vi "HOST_laser.vi"() -> ()   [LabVIEW 2018]
uses:
  <vilib>/rvi/interface/nirviOpenFPGA/nirviOpenFPGA.xnode
  <vilib>/rvi/interface/nirviMethod/nirviMethod.xnode
  <vilib>/FPGAPlugInAG/Dynamic/niLvFpga_Reset_Dynamic.vi
  <vilib>/FPGAPlugInAG/Dynamic/niLvFpga_Run_Dynamic.vi
  <vilib>/rvi/interface/nirviReadWriteControl/nirviReadWriteControl.xnode
  <vilib>/rvi/interface/nirviCloseFPGA/nirviCloseFPGA.xnode
  NiFpgaLv.dll
  <vilib>/Utility/error.llb/Error Cluster From Error Code.vi
  <vilib>/rvi/interface/Simulation/niFpgaSimulationCallBeginRW.vi
  <vilib>/rvi/errors/niLvFpgaAdjustHostInterfaceError.vi
  <vilib>/FPGAPlugInAG/Dynamic/niLvFpga_Close_Dynamic.vi
  FPGA Bitfiles/iCLNGNQI_FPGATarget_Target_OrC3no1FGAk.lvbitx
  <vilib>/FPGAPlugInAG/PXI-7841R/niLvFpga_Open_PXI-7841R.vi
  <vilib>/rvi/interface/common/dynamic/niFpgaDynamicAddResources.vi
  <vilib>/userdefined/High Color/nirio_resource_hc.ctl
panel:
  in  "Прошивка":bool
  in  "СТОП":bool
  out "Сбои":i32
  in  "resource name":T1="PXI1Slot6"
  in  "Сверочный массив":bool[][](array[boolean])=[[FALSE, FALSE, FALSE, FALSE, FALSE, TRUE, FALSE, TRUE], [FALSE, FALSE, FALSE, FALSE, FALSE, TRUE, FALSE, TRUE], [FALSE, FALSE, FALSE, FALSE, FALSE, FALSE, TRUE, TRUE], [FALSE, FALSE, FALSE, FALSE, FALSE, FALSE, TRUE, TRUE], [FALSE, FALSE, FALSE, FALSE, FALSE, FALSE, TRUE, TRUE], [FALSE, FALSE, FALSE, FALSE, FALSE, FALSE, TRUE, TRUE], [FALSE, FALSE, FALSE, FALSE, FALSE, TRUE, FALSE, TRUE], [TRUE, FALSE, FALSE, FALSE, FALSE, FALSE, FALSE, TRUE], [FALSE, TRUE, TRUE, FALSE, TRUE, FALSE, FALSE, TRUE]]
  in  "На чтение":bool[][](array[boolean])=[[FALSE, FALSE, FALSE, FALSE, FALSE, FALSE, FALSE, FALSE, FALSE, FALSE, FALSE, FALSE, FALSE, FALSE, FALSE, FALSE, FALSE, TRUE, FALSE, TRUE, FALSE, FALSE, FALSE, TRUE], [FALSE, FALSE, FALSE, FALSE, FALSE, FALSE, FALSE, FALSE, TRUE, FALSE, FALSE, FALSE, FALSE, FALSE, FALSE, FALSE, FALSE, TRUE, FALSE, TRUE, FALSE, FALSE, FALSE, TRUE], [FALSE, FALSE, FALSE, FALSE, FALSE, FALSE, FALSE, FALSE, FALSE, TRUE, FALSE, FALSE, FALSE, FALSE, FALSE, FALSE, FALSE, TRUE, FALSE, TRUE, FALSE, FALSE, FALSE, TRUE], [FALSE, FALSE, FALSE, FALSE, FALSE, FALSE, FALSE, FALSE, TRUE, TRUE, FALSE, FALSE, FALSE, FALSE, FALSE, FALSE, FALSE, TRUE, FALSE, TRUE, FALSE, FALSE, FALSE, TRUE], [FALSE, FALSE, FALSE, FALSE, FALSE, FALSE, FALSE, FALSE, FALSE, FALSE, TRUE, FALSE, FALSE, FALSE, FALSE, FALSE, FALSE, TRUE, FALSE, TRUE, FALSE, FALSE, FALSE, TRUE], [FALSE, FALSE, FALSE, FALSE, FALSE, FALSE, FALSE, FALSE, TRUE, FALSE, TRUE, FALSE, FALSE, FALSE, FALSE, FALSE, FALSE, TRUE, FALSE, TRUE, FALSE, FALSE, FALSE, TRUE], [FALSE, FALSE, FALSE, FALSE, FALSE, FALSE, FALSE, FALSE, FALSE, TRUE, TRUE, FALSE, FALSE, FALSE, FALSE, FALSE, FALSE, TRUE, FALSE, TRUE, FALSE, FALSE, FALSE, TRUE], [FALSE, FALSE, FALSE, FALSE, FALSE, FALSE, FALSE, FALSE, TRUE, TRUE, TRUE, FALSE, FALSE, FALSE, FALSE, FALSE, FALSE, TRUE, FALSE, TRUE, FALSE, FALSE, FALSE, TRUE], [FALSE, FALSE, FALSE, FALSE, FALSE, FALSE, FALSE, FALSE, FALSE, FALSE, FALSE, TRUE, FALSE, FALSE, FALSE, FALSE, FALSE, TRUE, FALSE, TRUE, FALSE, FALSE, FALSE, TRUE]]
  out "MISO":bool[](array[boolean])
  in  "MOSI":bool[](array[boolean])=[TRUE, TRUE, FALSE, FALSE, FALSE, FALSE, FALSE, TRUE, FALSE, FALSE, FALSE, FALSE, TRUE, TRUE, FALSE, TRUE, FALSE, FALSE, FALSE, FALSE, FALSE, FALSE, FALSE, FALSE]
  in  "N (24/16)":i32=16
  # "Ковёр"
  # "0"
  # "1"
  # "2"
  # "3"
  # "4"
  # "5"
  # "6"
  # "7"
  # "0"
  # "1"
  # "2"
  # "3"
  # "4"
  # "5"
  # "6"
  # "7"
  # "0"
  # "1"
  # "2"
  # "3"
  # "4"
  # "5"
  # "6"
  # "7"
  # "LNG"
  # "0"
  # "1"
  # "2"
  # "3"
  # "4"
  # "5"
  # "6"
  # "7"
  # "0"
  # "1"
  # "2"
  # "3"
  # "4"
  # "5"
  # "6"
  # "7"
  # "0"
  # "1"
  # "2"
  # "3"
  # "4"
  # "5"
  # "6"
  # "7"
  # "ADDRESS"
  # "DATA"
  # "OPCODE"
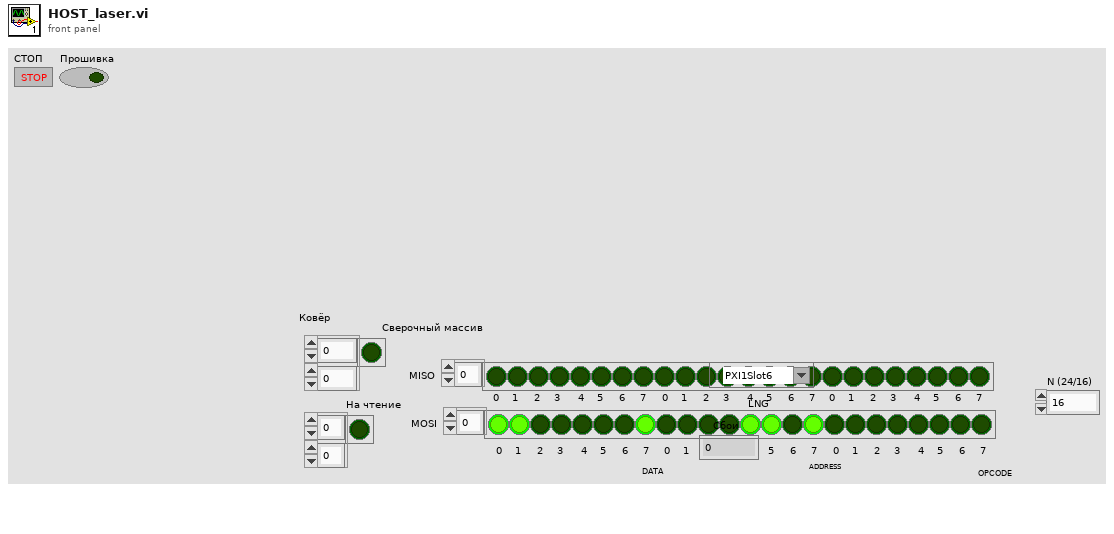
[diagram p1: front panel]
types:
  T1 = typedef "nirio_resource_hc.ctl" = tag
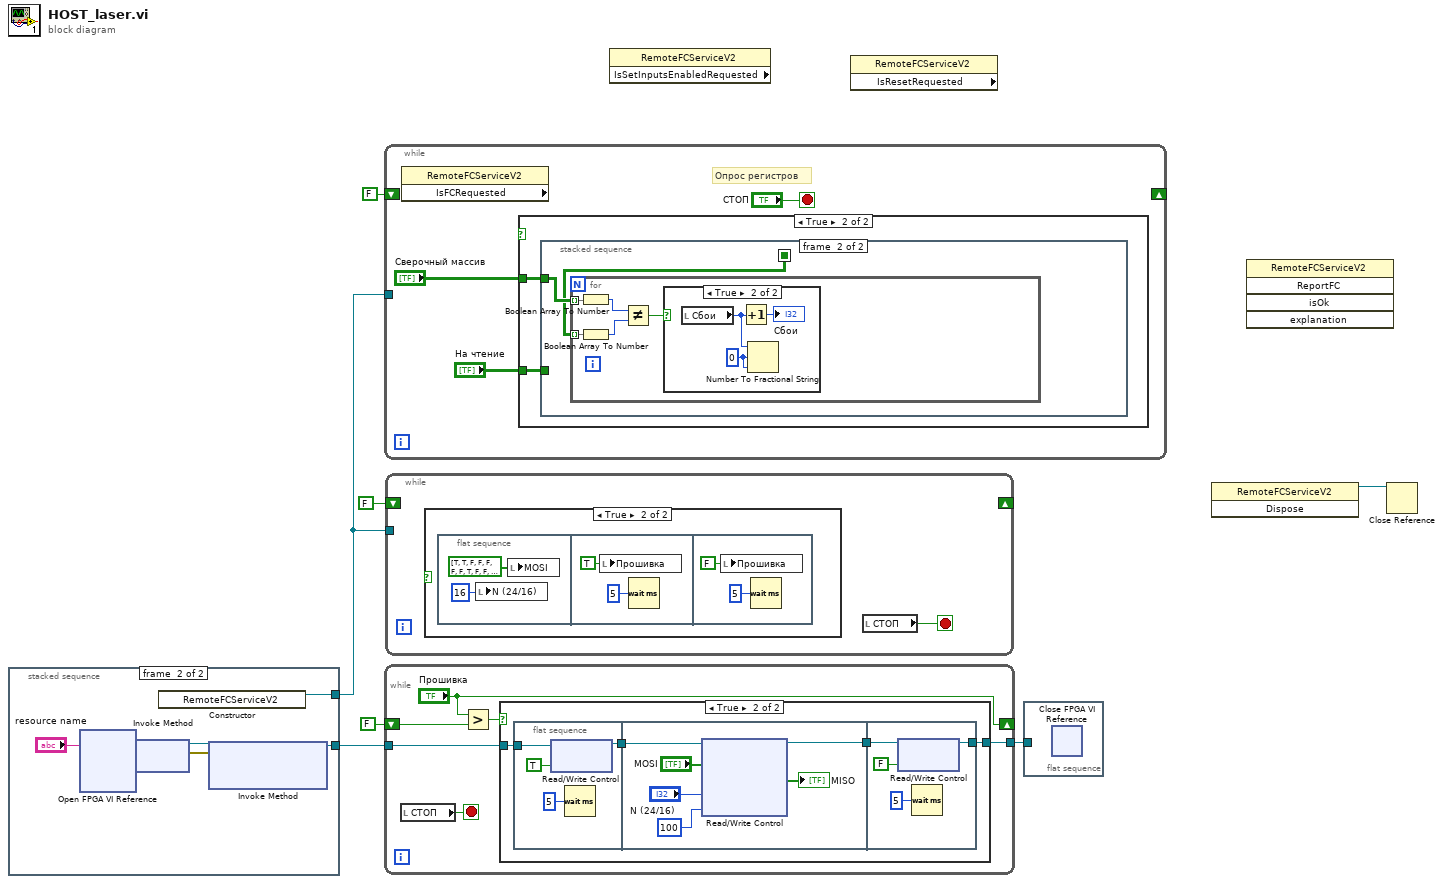
[diagram p0: block diagram]
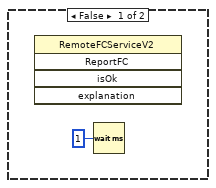
[diagram p2: hidden frame]
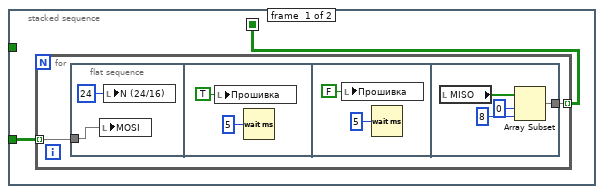
[diagram p3: hidden frame]
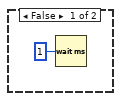
[diagram p5: hidden frame]
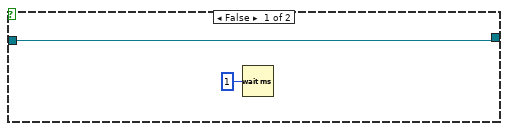
[diagram p6: hidden frame]
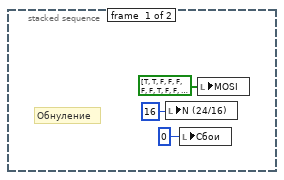
[diagram p7: hidden frame]
diagram:
  n1 = stacked-sequence {
    tunnel: [_ w12] -> w4
    tunnel: [_ w11] -> w3
    frame #0 {
      # "Обнуление"
      n2 = local write "N (24/16)"(16 ("N (24/16)")) -> ()
      n3 = local write "Сбои"(0 ("Сбои")) -> ()
      n4 = local write "MOSI"(bool[] [TRUE, TRUE, FALSE, FALSE, FALSE, FALSE, FALSE, TRUE, FALSE, FALSE, FALSE, FALSE, TRUE, TRUE, FALSE, TRUE, FALSE, FALSE, FALSE, FALSE, FALSE, FALSE, FALSE, FALSE] ("MOSI")) -> ()
    }
    frame #1 {
      n5 = xnode "Open FPGA VI Reference"("resource name"="resource name") -> ("FPGA VI Reference Out"=w13:refnum<k20>, "error out"=w15:errorcluster)  [unwired: 1 in]
      n6 = xnode "Invoke Method"("FPGA VI Reference In"=w13, "error in"=w15) -> ("FPGA VI Reference Out"=w16:refnum<k20>, "error out"=w14:errorcluster)
      n7 = constructor class="RemoteFCServiceV2"() -> (reference out=w11:refnum<k24>)  [unwired: 3 in, 2 out]
      n8 = xnode "Invoke Method"("FPGA VI Reference In"=w16, "error in"=w14) -> ("FPGA VI Reference Out"=w12:refnum<k20>)  [unwired: 1 in, 1 out]
    }
  }
  n9 = while {
    tunnel: w3 -> [_]
    shift-right: _ -> [_]
    shift-left: FALSE -> [_]
    stop <- "СТОП" stop-if-true
    # "Опрос регистров"
    n10 = property class="RemoteFCServiceV2" props=["IsFCRequested"]() -> ()  [unwired: 2 in, 3 out]
    n11 = case shown="True" {
      selector: _ -> [_ _]
      tunnel: "Сверочный массив" -> [_ w22]
      tunnel: "На чтение" -> [_ w23]
      frame False {
        n12 = invoke class="RemoteFCServiceV2" method="ReportFC"() -> ()  [unwired: 5 in, 5 out]
        n13 = Wait (ms)(milliseconds to wait=u32 1) -> ()  [unwired: 1 out]
      }
      frame True {
        n14 = stacked-sequence {
          seq-local: [w25 _] -> [_ w38]
          tunnel: w23 -> [w24 _]
          tunnel: w22 -> [_ w39]
          frame #0 {
            n15 = for {
              tunnel: [w27] -> w25 mode=indexing
              tunnel: w24 -> [w26] mode=indexing
              n16 = flat-sequence {
                tunnel: w26 -> [w28]
                tunnel: [w34] -> w27
                frame #0 {
                  n17 = local write "MOSI"(w28) -> ()
                  n18 = local write "N (24/16)"(24 ("N (24/16)")) -> ()
                }
                frame #1 {
                  n19 = local write "Прошивка"(TRUE ("Прошивка")) -> ()
                  n20 = Wait (ms)(milliseconds to wait=u32 5) -> ()  [unwired: 1 out]
                }
                frame #2 {
                  n21 = local write "Прошивка"(FALSE ("Прошивка")) -> ()
                  n22 = Wait (ms)(milliseconds to wait=u32 5) -> ()  [unwired: 1 out]
                }
                frame #3 {
                  n23 = local read "MISO"() -> (w37:bool[])
                  n24 = Array Subset(array=w37, index=0, length=8) -> (w34:bool[])
                }
              }
            }
          }
          frame #1 {
            n25 = for {
              tunnel: w39 -> [w44] mode=indexing
              tunnel: w38 -> [w43] mode=indexing
              n26 = Boolean Array To Number(Boolean array=w44) -> (number=w42:u32)
              n27 = Boolean Array To Number(Boolean array=w43) -> (number=w41:u32)
              n28 = Not Equal?(x=w42, y=w41) -> (x != y?=w40:bool)
              n29 = case shown="True" w40 {
                frame False {
                }
                frame True {
                  w47 = i16 0 ("width (-)")
                  n30 = local read "Сбои"() -> (w45:i32)
                  n31 = Increment(x=w45) -> (x+1=→"Сбои":i32)
                  n32 = Number To Fractional String(number=w45, width (-)=w47, precision (6)=w47) -> ()  [unwired: 1 in, 1 out]
                }
              }
            }
          }
        }
      }
    }
  }
  n33 = while {
    tunnel: w4 -> [w53]
    tunnel: [w52] -> w7
    shift-right: ["Прошивка"] -> _
    shift-left: FALSE ("Прошивка") -> [w50]
    stop <- w51 stop-if-true
    n34 = local read "СТОП"() -> (w51:bool)
    n35 = Greater?(x="Прошивка", y=w50) -> (0:w48:bool)
    n36 = case shown="True" w48 {
      tunnel: w53 -> [w54 w59]
      tunnel: [w54 w56] -> w52
      frame False {
        n37 = Wait (ms)(milliseconds to wait=u32 1) -> ()  [unwired: 1 out]
      }
      frame True {
        n38 = flat-sequence {
          tunnel: w59 -> [w63]
          tunnel: [w60] -> w58
          tunnel: w58 -> [w67]
          tunnel: [w66] -> w57
          tunnel: w57 -> [w71]
          tunnel: [w70] -> w56
          frame #0 {
            n39 = xnode "Read/Write Control"("FPGA VI Reference In"=w63, "Регистр"=TRUE) -> ("FPGA VI Reference Out"=w60:refnum<k20>)  [unwired: 1 in, 1 out]
            n40 = Wait (ms)(milliseconds to wait=u32 5) -> ()  [unwired: 1 out]
          }
          frame #1 {
            n41 = xnode "Read/Write Control"("FPGA VI Reference In"=w67, "MOSI"="MOSI", "N (24/16)"="N (24/16)", "Count(Ticks)"=u16 100) -> ("FPGA VI Reference Out"=w66:refnum<k20>, "MISO"=→"MISO":bool[])  [unwired: 1 in, 1 out]
          }
          frame #2 {
            n42 = xnode "Read/Write Control"("FPGA VI Reference In"=w71, "Регистр"=FALSE) -> ("FPGA VI Reference Out"=w70:refnum<k20>)  [unwired: 1 in, 1 out]
            n43 = Wait (ms)(milliseconds to wait=u32 5) -> ()  [unwired: 1 out]
          }
        }
      }
    }
  }
  n44 = while {
    shift-right: _ -> [_]
    shift-left: FALSE ("POWER_LNG") -> [_]
    tunnel: w3 -> [_]
    stop <- w74 stop-if-true
    n45 = case shown="True" {
      selector: _ -> [_ _]
      frame False {
        n46 = Wait (ms)(milliseconds to wait=u32 1) -> ()  [unwired: 1 out]
      }
      frame True {
        n47 = flat-sequence {
          frame #0 {
            n48 = local write "N (24/16)"(16 ("N (24/16)")) -> ()
            n49 = local write "MOSI"(bool[] [TRUE, TRUE, FALSE, FALSE, FALSE, FALSE, FALSE, TRUE, FALSE, FALSE, FALSE, FALSE, TRUE, TRUE, FALSE, TRUE, FALSE, FALSE, FALSE, FALSE, FALSE, FALSE, FALSE, FALSE] ("MOSI")) -> ()
          }
          frame #1 {
            n50 = local write "Прошивка"(TRUE ("Прошивка")) -> ()
            n51 = Wait (ms)(milliseconds to wait=u32 5) -> ()  [unwired: 1 out]
          }
          frame #2 {
            n52 = local write "Прошивка"(FALSE ("Прошивка")) -> ()
            n53 = Wait (ms)(milliseconds to wait=u32 5) -> ()  [unwired: 1 out]
          }
        }
      }
    }
    n54 = local read "СТОП"() -> (w74:bool)
  }
  n55 = property class="RemoteFCServiceV2" props=["IsSetInputsEnabledRequested"]() -> ()  [unwired: 2 in, 3 out]
  n56 = property class="RemoteFCServiceV2" props=["IsResetRequested"]() -> ()  [unwired: 2 in, 3 out]
  n57 = flat-sequence {
    tunnel: w7 -> [_]
    frame #0 {
      n58 = xnode "Close FPGA VI Reference"() -> ()  [unwired: 2 in, 1 out]
    }
  }
  n59 = invoke class="RemoteFCServiceV2" method="Dispose"() -> (reference out=w2:refnum<k24>)  [unwired: 3 in, 2 out]
  n60 = invoke class="RemoteFCServiceV2" method="ReportFC"() -> ()  [unwired: 5 in, 5 out]
  n61 = Close Reference(reference=w2) -> ()  [unwired: 1 in, 1 out]
